vi "Configure Major Frame.vi"(8 "Error in (no error)":errorcluster, 9 "Minor Frame IDs":u8[](array[numeric]), 10 "Major Frame ID in":u8=1, 11 "Module Handle in":u32) -> (0 "Error out":errorcluster, 2 "Major Frame ID out":u8=1, 3 "Module Handle out":u32)   [LabVIEW 2020, in "AIM MIL-STD-1553 Hardware API.lvlib"]
uses:
  AIM MIL-STD-1553 Hardware API.lvlib
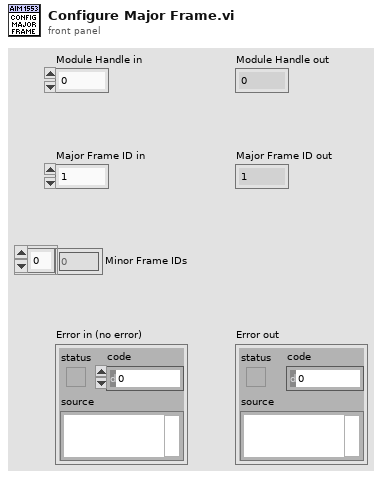
[diagram p1: front panel]
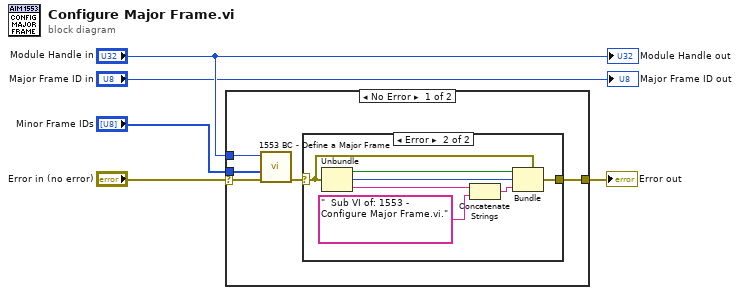
[diagram p0: block diagram]
diagram:
  n1 = case shown="No Error" "Error in (no error)" {
    tunnel: "Minor Frame IDs" -> [w6 _]
    selector: "Error in (no error)" -> [w10 w19]
    tunnel: [w8 w19] -> w5
    tunnel: "Module Handle in" -> [w7 _]
    frame No Error {
      n2 = call <instrlib>:"1553 BC - Define a Major Frame.vi"("Error In (none)"=w10, "Frame List"=w6, "Module Handle"=w7) -> ("Error Out"=w9:errorcluster)  [unwired: 7 in, 1 out]
      n3 = case shown="Error" w9 {
        selector: w9 -> [w11 w18]
        tunnel: [w11 w15] -> w8
        frame No Error {
        }
        frame Error {
          n4 = Unbundle(w18) -> ("status"=w16:bool, "code"=w17:i32, "source"=w14:string)
          n5 = Concatenate Strings(w14, "  Sub VI of: 1553 - Configure Major Frame.vi.") -> (w13:string)
          n6 = Bundle(cluster=w18, "status"=w16, "code"=w17, "source"=w13) -> (w15:errorcluster)
        }
      }
    }
    frame Error {
    }
  }
  "Error out" <- w5
  "Module Handle out" <- "Module Handle in"
  "Major Frame ID out" <- "Major Frame ID in"
